vi "task.identifier_lua.vi"(5 "LuaVIEW reference":T1) -> (15 "error out":errorcluster)   [LabVIEW 2012]
doc: "Returns the calling task's own identifier. A task might want to know its own identifier in order to format more easily interpretable error or log messages, or to be able to pass its identifier to a different task so as to set up for bidirectional messaging.\n\nIt is possible to assign a specific identifier to a task by using the \"--#identifier\" preprocessor keyword as part of its main script. This prevents additional task scripts with the same identifier from being started. If there is no problem with starting multiple instances of a task script, the \"--#identifier\" keyword can be omitted. In that case a unique number is assigned as identifier to each instance.\nResults:\nstr:identifier\nErrors:\nFunction must be called from a task context but was not."
uses:
  typedefs/t_LuaVIEW Reference.ctl
  typedefs/t_LuaVIEW Task State Methods.ctl
  subvis/private/LuaVIEW Push (string).vi
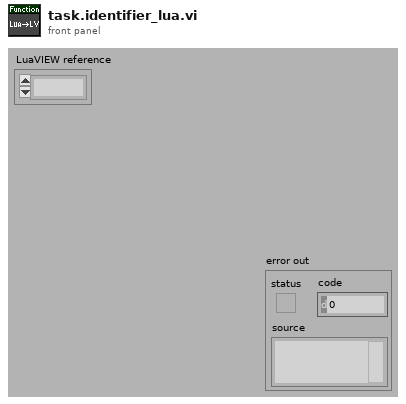
[diagram p1: front panel]
types:
  T1 = typedef "t_LuaVIEW Reference.ctl" = refnum<k1>
  T2 = typedef "t_LuaVIEW Task State Methods.ctl" = enum16{"cleanup", "set initial", "set mode", "set active mode", "set error", "get task info", "get script info", "set signal", "clear signal", "test handled", "test delegated", "test signal", "handle signal", "delegate signal", "allow signal", "disallow signal", "disallow all", "signals?", "delegated signals?", "protection++", "protection--", "protection=0", "message", "next message", "pop message", "message available?", "force stop", "set swap preps", "apply swap preps"}
  T3 = typedef "t_LuaVIEW Task State Pane.ctl" = refnum<vi>
  T4 = typedef "LuaVIEW Task Info.ctl" = cluster{"main script":string, "identifier":string, "class":string, "description":string, "mode":T5, "handler":string, "LuaVIEW reference":T1, "scripts":i32, "hide":bool, "active":bool, "error msg":string, "defer":bool, "launch":enum16{"asynchronous", "manual", "synchronous"}, "main path valid":bool, "start time":dbl, "swap time":dbl, "task VI":refnum<vi>, "prefsys":enum32{"invalid execution system", "user interface", "standard", "instrument i/o", "data acquisition", "other 1", "other 2", "same as caller"}, "priority":enum32{"invalid priority", "background priority", "normal priority", "above normal priority", "high priority", "time critical priority", "subroutine"}, "signal flags":u32, "allow mask":u32, "handle mask":u32, "disallow manual":bool}
  T5 = typedef "t_LuaVIEW Task Modes.ctl" = enum16{"initializing", "running", "executing", "paused", "error", "swapping"}
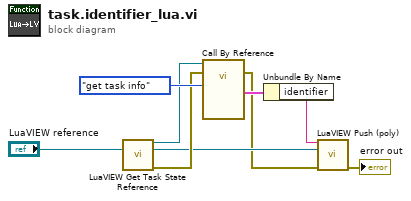
[diagram p0: block diagram]
diagram:
  n1 = call "LuaVIEW Get Task State Reference.vi"("LuaVIEW reference in"="LuaVIEW reference") -> ("task state reference"=w7:T3, "LuaVIEW reference out"=w5:T1, "error out"=w6:errorcluster)  [unwired: 12 in]
  n2 = call-by-ref "?"(reference=w7, error in=w6, "method"=t_LuaVIEW_Task_State_Methods."get task info") -> (error out=w3:errorcluster, "task info {get task info}"=w8:T4)  [unwired: 10 in, 5 out]
  n3 = Unbundle By Name(w8) -> ("identifier"=w4:string)
  n4 = call-poly "LuaVIEW Push (poly).vi"("string"=w4, "LuaVIEW reference in"=w5, "error in (no error)"=w3) -> ("error out"=→"error out":errorcluster)  [unwired: 11 in, 1 out]
